vi "NetworkVd(SubVI).vi"(1 "Array":dbl[](array[numeric])) -> (0 "Numeric":dbl)   [LabVIEW 2021]
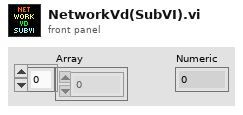
[diagram p1: front panel]
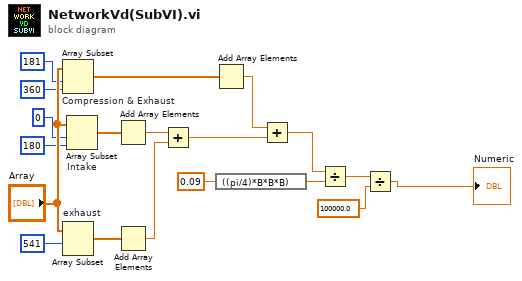
[diagram p0: block diagram]
diagram:
  n1 = Array Subset "Compression & Exhaust"(array="Array", index=181, length=360) -> (w11:dbl[])
  n2 = Array Subset "exhaust"(array="Array", index=541) -> (w8:dbl[])  [unwired: 1 in]
  n3 = Array Subset "Intake"(array="Array", index=0, length=180) -> (w7:dbl[])
  n4 = Add Array Elements(numeric array=w7) -> (sum=w9:dbl)
  n5 = Add Array Elements(numeric array=w8) -> (sum=w10:dbl)
  n6 = Add(x=w9, y=w10) -> (x+y=w17:dbl)
  n7 = Add Array Elements(numeric array=w11) -> (sum=w19:dbl)
  n8 = expression code="((pi/4)*B*B*B)"(0.09) -> (w14:dbl)
  n9 = Add(x=w19, y=w17) -> (x+y=w18:dbl)
  n10 = Divide(x=w18, y=w14) -> (x/y=w13:dbl)
  n11 = Divide(x=w13, y=100000.0) -> (x/y=→"Numeric":dbl)
